vi "App_Main 2.vi"() -> ()   [LabVIEW 2015, in "Application 2.lvlib"]
uses:
  Application 2.lvlib
  Cloud Server/Data Def/Server_Error Handle Method.ctl
  Data Def/App_Subpanel Name.ctl
  Data Def/App_User Event Data.ctl
  Data Def/App_Main Loop Queue Data.ctl
  Data Def/App_Tips Data.ctl
  Cloud Server/Cloud Server.lvlib
panel:
  out "Time":timestamp format="%<%H:%M:%S>T"
  out "Connection?":bool
  out "User Name":string
  out "Login?":bool
  out "Tips":string
  in  "Stop":bool caption="Power"
  in  "Home":bool caption="Menu"
  # "Smart ECG Client"
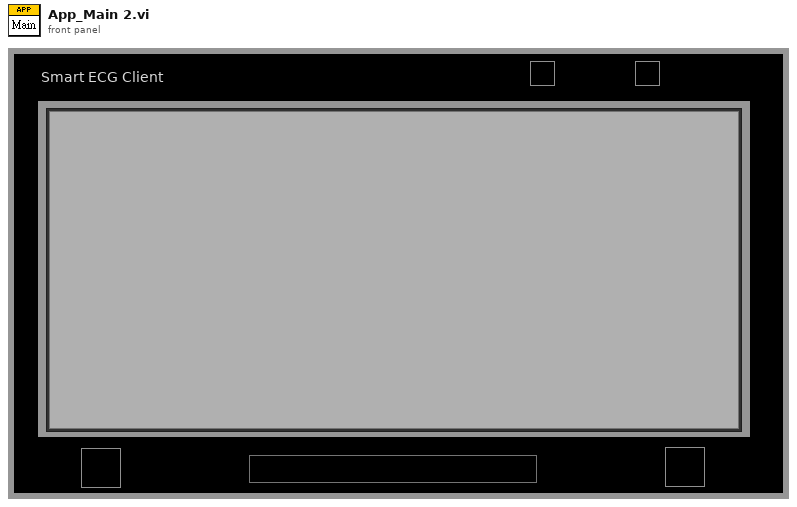
[diagram p1: front panel]
types:
  T1 = typedef "Cloud Server.lvlib/Server_Error Handle Method.ctl" = enum16{"Initialize", "Get Queue Ref.", "Enqueue", "Insert", "Flush", "Release"}
  T2 = typedef "Application 2.lvlib/App_User Event Data.ctl" = cluster{"Command":string, "Data":variant}
  T3 = typedef "Application 2.lvlib/App_Subpanel Name.ctl" = enum16{"Main", "Menu", "User Registering", "User Setting", "Monitor", "Traning Mode", "Query Data", "Connect Setting"}
  T4 = typedef "Application 2.lvlib/App_Main Loop Queue Data.ctl" = cluster{"Command":string, "Data":variant}
  T5 = typedef "Application 2.lvlib/App_Main Data.ctl" = cluster{"VI Refnum":refnum<vi>, "Subpanel":refnum<vi>, "Connection ID":refnum<k5>, "Meta data":T6[], "Main Queue":T8, "User Data":T9}
  T6 = typedef "stm_MetaElement.ctl" = cluster{"Name":T7}
  T7 = typedef "stm_MetaDataElement.ctl" = string
  T8 = typedef "Application 2.lvlib/App_Main Queue.ctl" = cluster{"Main Loop Queue":refnum<queue>}
  T9 = typedef "User Data.ctl" = cluster{"Name":string, "Email":string, "Phone Number":string, "User Picture":u32[][], "Last Login Time":timestamp}
  T10 = typedef "Application 2.lvlib/App_Tips Data.ctl" = cluster{"Tips":string, "BG Color":u32}
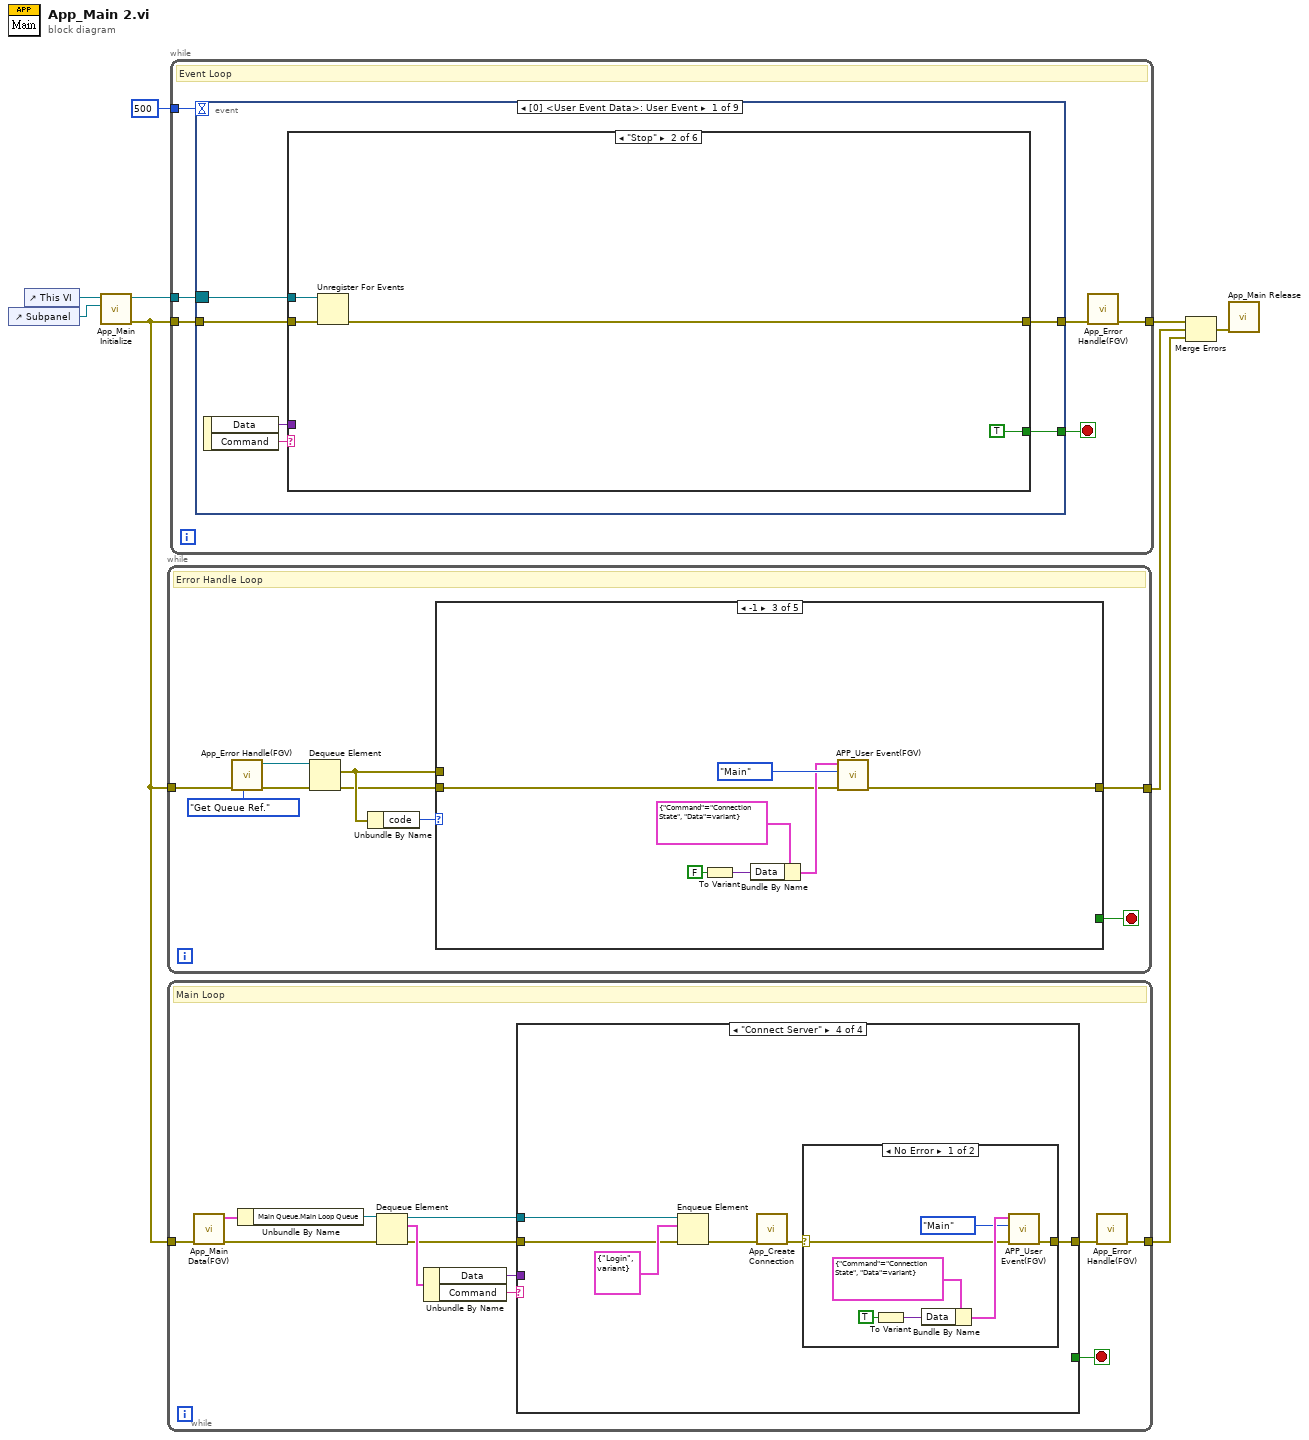
[diagram p0: block diagram]
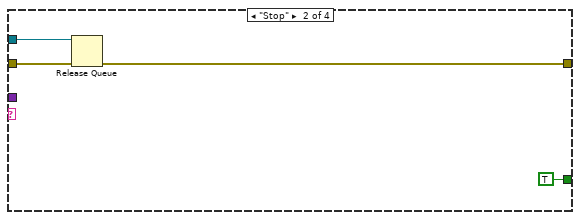
[diagram p3: hidden frame]
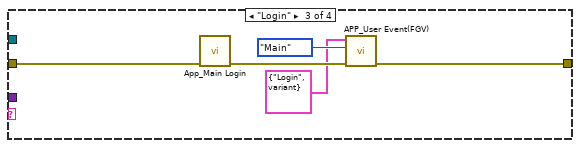
[diagram p4: hidden frame]
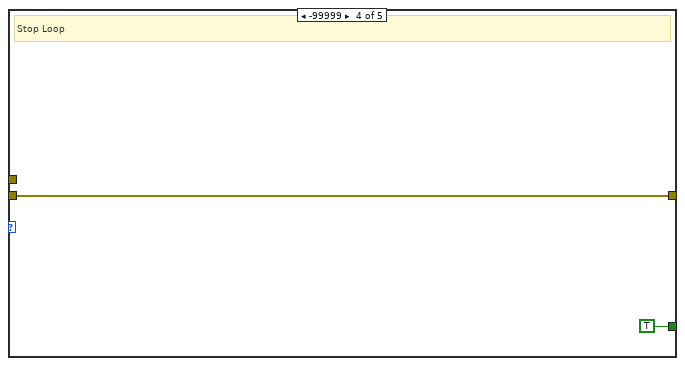
[diagram p8: hidden frame]
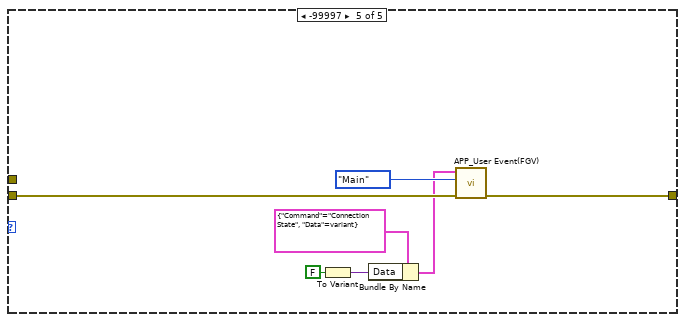
[diagram p9: hidden frame]
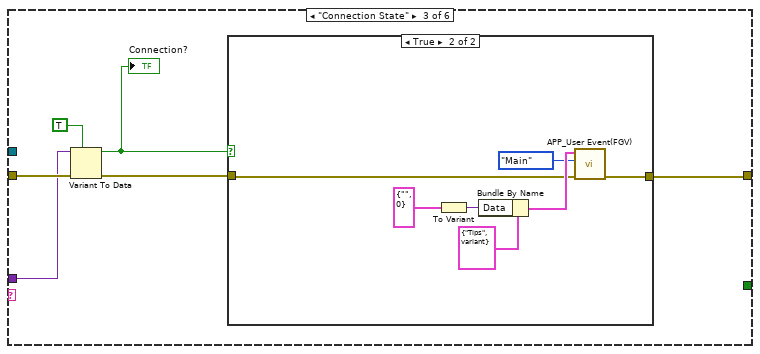
[diagram p11: hidden frame]
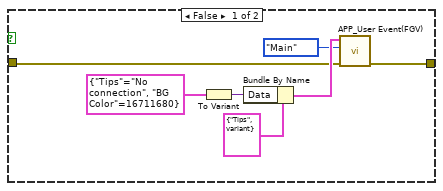
[diagram p12: hidden frame]
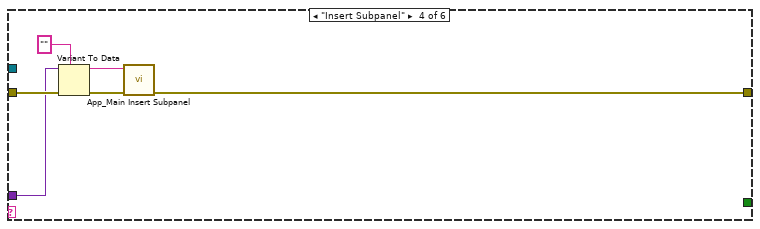
[diagram p13: hidden frame]
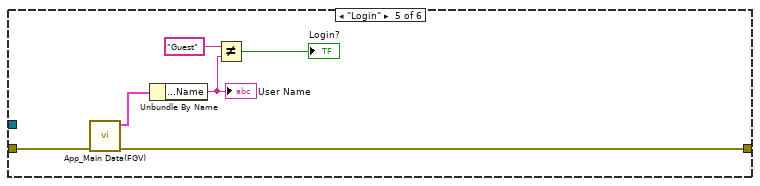
[diagram p14: hidden frame]
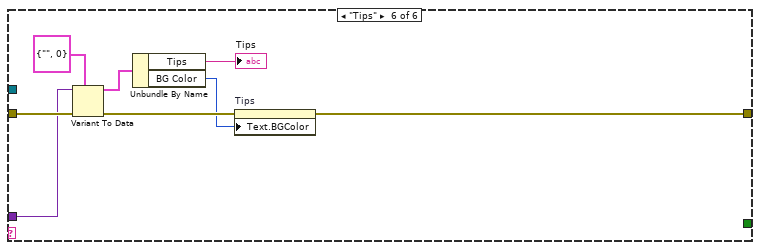
[diagram p15: hidden frame]
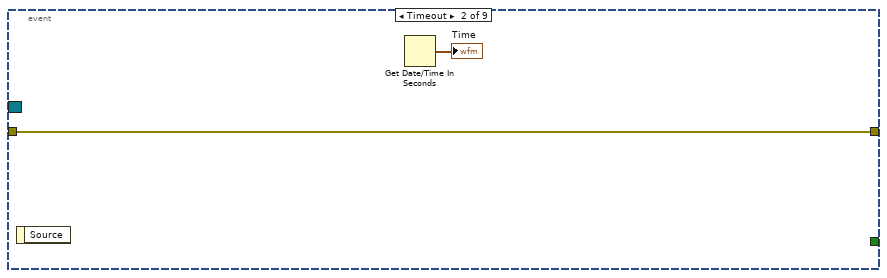
[diagram p16: hidden frame]
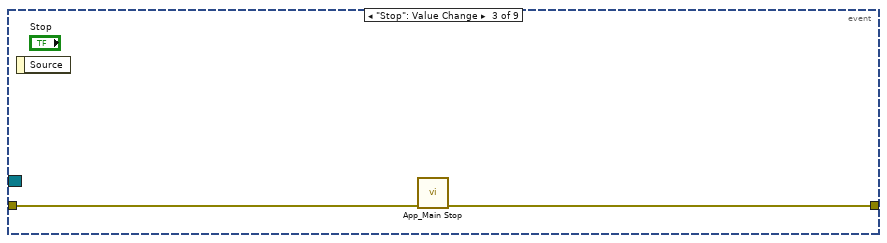
[diagram p17: hidden frame]
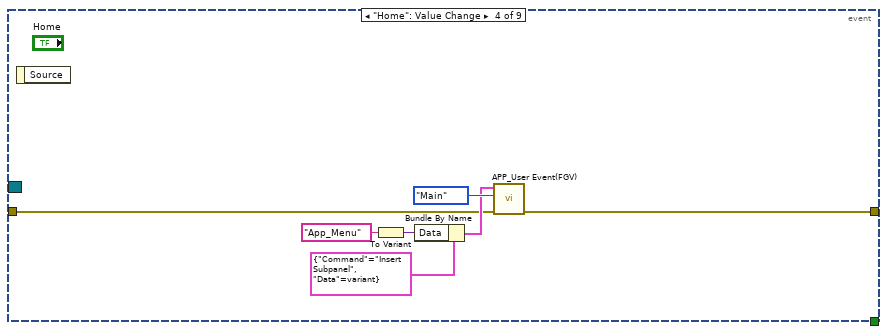
[diagram p18: hidden frame]
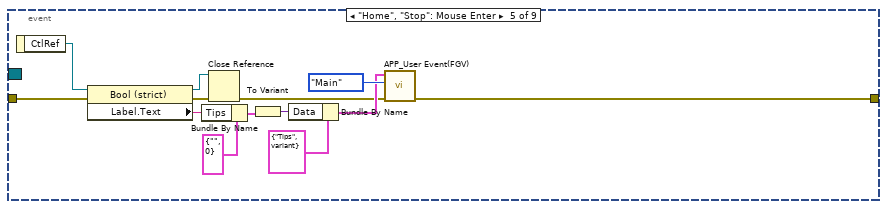
[diagram p19: hidden frame]
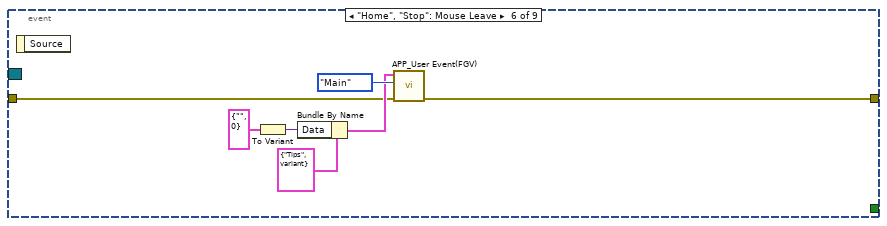
[diagram p20: hidden frame]
diagram:
  n1 = control-ref of="Subpanel"() -> (w7:refnum<vi>)
  n2 = control-ref of="This VI"() -> (w9:refnum<vi>)
  n3 = call "App_Main Initialize.vi"("Subpanel"=w7, "VI Reference"=w9) -> ("error out"=w2:errorcluster, "Event Registration Refnum"=w8:refnum<event-registration>)  [unwired: 8 in]
  n4 = while {
    tunnel: w2 -> [w18]
    tunnel: [w10] -> w4
    stop <- w11 stop-if-true
    # "Error Handle Loop"
    n5 = call "App_Error Handle(FGV).vi"("Error Handle Method(Enqueue)"=Server_Error_Handle_Method."Get Queue Ref.", "error in"=w18) -> ("error out"=w16:errorcluster, "Queue Ref."=w15:refnum<queue>)  [unwired: 8 in]
    n6 = Dequeue Element(queue=w15, error in (no error)=w16) -> (element=w13:errorcluster, error out=w12:errorcluster)  [unwired: 1 in, 2 out]
    n7 = Unbundle By Name(w13) -> ("code"=w14:i32)
    n8 = case shown="-1" w14 {
      tunnel: w13 -> [_ _ _ _ _]
      tunnel: w12 -> [w19 w20 w22 w28 w35]
      tunnel: [_ _ _ TRUE _] -> w11
      tunnel: [w19 w20 w21 w28 w30] -> w10
      frame Default {
        # "Undefine error"
      }
      frame 0 {
        # "No error"
      }
      frame -1 {
        n9 = To Variant(anything=FALSE) -> (Variant=w25:variant)
        n10 = Bundle By Name(cluster=T2 {"Command"="Connection State", "Data"=variant} ("User Event Data"), "Data"=w25) -> (w23:T2)
        n11 = call "APP_User Event(FGV).vi"("error in"=w22, "Subpanel Name"=App_Subpanel_Name."Main", "User Event Data"=w23) -> ("error out"=w21:errorcluster)  [unwired: 7 in, 1 out]
      }
      frame -99999 {
        # "Stop Loop"
      }
      frame -99997 {
        n12 = To Variant(anything=FALSE) -> (Variant=w33:variant)
        n13 = Bundle By Name(cluster=T2 {"Command"="Connection State", "Data"=variant} ("User Event Data"), "Data"=w33) -> (w31:T2)
        n14 = call "APP_User Event(FGV).vi"("error in"=w35, "Subpanel Name"=App_Subpanel_Name."Main", "User Event Data"=w31) -> ("error out"=w30:errorcluster)  [unwired: 7 in, 1 out]
      }
    }
  }
  n15 = while {
    tunnel: w2 -> [w48]
    tunnel: [w39] -> w1
    stop <- w37 stop-if-true
    # "Main Loop"
    n16 = call "App_Main Data(FGV).vi"("error in"=w48) -> ("error out"=w46:errorcluster, "Main Data Out"=w47:T5)  [unwired: 9 in]
    n17 = Unbundle By Name(w47) -> ("Main Queue.Main Loop Queue"=w45:refnum<queue>)
    n18 = Dequeue Element(queue=w45, error in (no error)=w46) -> (queue out=w38:refnum<queue>, element=w44:T4, error out=w41:errorcluster)  [unwired: 1 in, 1 out]
    n19 = Unbundle By Name(w44) -> ("Data"=w42:variant, "Command"=w43:string)
    n20 = case shown="\"Connect Server\"" w43 {
      tunnel: w42 -> [_ _ _ _]
      tunnel: w41 -> [w49 w53 w58 w61]
      tunnel: [w49 w51 w54 w63] -> w40
      tunnel: w38 -> [_ w52 _ w59]
      tunnel: [_ TRUE _ _] -> w37
      frame Default {
      }
      frame "Stop" {
        n21 = Release Queue(queue=w52, error in (no error)=w53) -> (error out=w51:errorcluster)  [unwired: 1 in, 2 out]
      }
      frame "Login" {
        n22 = call "App_Main Login.vi"("error in"=w58) -> ("error out"=w56:errorcluster)  [unwired: 10 in]
        n23 = call "APP_User Event(FGV).vi"("error in"=w56, "Subpanel Name"=App_Subpanel_Name."Main", "User Event Data"=T2 {"Command"="Login", "Data"=variant}) -> ("error out"=w54:errorcluster)  [unwired: 7 in, 1 out]
      }
      frame "Connect Server" {
        n24 = Enqueue Element(queue=w59, element=T4 {"Command"="Login", "Data"=variant}, error in (no error)=w61) -> (error out=w60:errorcluster)  [unwired: 1 in, 2 out]
        n25 = call "App_Create Connection.vi"("error in"=w60) -> ("error out"=w64:errorcluster)  [unwired: 10 in]
        n26 = case shown="No Error" w64 {
          selector: w64 -> [w66 w72]
          tunnel: [w65 w72] -> w63
          frame No Error {
            n27 = To Variant(anything=TRUE) -> (Variant=w69:variant)
            n28 = Bundle By Name(cluster=T2 {"Command"="Connection State", "Data"=variant} ("User Event Data"), "Data"=w69) -> (w71:T2)
            n29 = call "APP_User Event(FGV).vi"("error in"=w66, "Subpanel Name"=App_Subpanel_Name."Main", "User Event Data"=w71) -> ("error out"=w65:errorcluster)  [unwired: 7 in, 1 out]
          }
          frame Error {
          }
        }
      }
    }
    n30 = call "App_Error Handle(FGV).vi"("error in"=w40) -> ("error out"=w39:errorcluster)  [unwired: 9 in, 1 out]
  }
  n31 = while {
    tunnel: w2 -> [w77]
    tunnel: w8 -> [w78]
    tunnel: [w74] -> w5
    tunnel: 500 -> [w73]
    stop <- w76 stop-if-true
    # "Event Loop"
    n32 = event shown="[0] <User Event Data>: User Event" {
      selector: w78 -> [w81 _ _ _ _ _ _ _ _]
      dyn-events: _ -> [_ _ _ _ _ _ _ _ _]
      timeout: w73 -> [_ _ _ _ _ _ _ _ _]
      tunnel: w77 -> [w82 w130 w133 w135 w153 w156 w164 w169 w183]
      tunnel: [w80 w130 w132 w134 w144 w155 w163 w168 w182] -> w75
      tunnel: [w79 _ _ _ _ _ _ _ _] -> w76
      event User Event {
        n33 = event-data() -> ("Data"=w83:variant, "Command"=w84:string)  [unwired: 1 in]
        n34 = case shown="\"Stop\"" w84 {
          tunnel: w83 -> [_ _ w94 w114 _ w128]
          tunnel: w82 -> [w85 w89 w95 w115 w121 w129]
          tunnel: w81 -> [_ w88 _ _ _ _]
          tunnel: [w85 w87 w90 w110 w119 w126] -> w80
          tunnel: [_ TRUE _ _ _ _] -> w79
          frame Default {
          }
          frame "Stop" {
            n35 = Unregister For Events(event registration refnum=w88, error in=w89) -> (error out=w87:errorcluster)
          }
          frame "Connection State" {
            n36 = Variant To Data(error in=w95, type=TRUE, Variant=w94) -> (data=w91:bool, error out=w92:errorcluster)
            "Connection?" <- w91
            n37 = case shown="True" w91 {
              tunnel: w92 -> [w97 w104]
              tunnel: [w96 w103] -> w90
              frame False {
                n38 = To Variant(anything=T10 {"Tips"="No connection", "BG Color"=16711680} ("Tips Data")) -> (Variant=w100:variant)
                n39 = Bundle By Name(cluster=T2 {"Command"="Tips", "Data"=variant} ("User Event Data"), "Data"=w100) -> (w101:T2)
                n40 = call "APP_User Event(FGV).vi"("error in"=w97, "Subpanel Name"=App_Subpanel_Name."Main", "User Event Data"=w101) -> ("error out"=w96:errorcluster)  [unwired: 7 in, 1 out]
              }
              frame True {
                n41 = To Variant(anything=T10 {"Tips"="", "BG Color"=0} ("Tips Data")) -> (Variant=w107:variant)
                n42 = Bundle By Name(cluster=T2 {"Command"="Tips", "Data"=variant} ("User Event Data"), "Data"=w107) -> (w108:T2)
                n43 = call "APP_User Event(FGV).vi"("error in"=w104, "Subpanel Name"=App_Subpanel_Name."Main", "User Event Data"=w108) -> ("error out"=w103:errorcluster)  [unwired: 7 in, 1 out]
              }
            }
          }
          frame "Insert Subpanel" {
            n44 = Variant To Data(error in=w115, type="", Variant=w114) -> (data=w111:string, error out=w112:errorcluster)
            n45 = call "App_Main Insert Subpanel.vi"("error in"=w112, "VI Name"=w111) -> ("error out"=w110:errorcluster)  [unwired: 9 in]
          }
          frame "Login" {
            n46 = call "App_Main Data(FGV).vi"("error in"=w121) -> ("error out"=w119:errorcluster, "Main Data Out"=w120:T5)  [unwired: 9 in]
            n47 = Unbundle By Name(w120) -> ("User Data.Name"=w118:string)
            "User Name" <- w118
            n48 = Not Equal?(x="Guest", y=w118) -> (x != y?=→"Login?":bool)
          }
          frame "Tips" {
            n49 = Variant To Data(error in=w129, type=T10 {"Tips"="", "BG Color"=0} ("Tips Data"), Variant=w128) -> (data=w124:T10, error out=w127:errorcluster)
            n50 = Unbundle By Name(w124) -> ("Tips"=→"Tips":string, "BG Color"=w122:u32)
            n51 = property on="Tips" class="Str"(error in=w127, "Text.BGColor"=w122) -> (error out=w126:errorcluster)  [unwired: 1 in, 1 out]
          }
        }
      }
      event Timeout {
        n52 = event-data() -> ()  [unwired: 1 in, 1 out]
        n53 = Get Date/Time In Seconds() -> (seconds since 1Jan1904=→"Time":timestamp)
      }
      event "Stop": Value Change {
        n54 = event-data() -> ()  [unwired: 1 in, 1 out]
        n55 = call "App_Main Stop.vi"("error in"=w133) -> ("error out"=w132:errorcluster)  [unwired: 10 in]
      }
      event "Home": Value Change {
        n56 = event-data() -> ()  [unwired: 1 in, 1 out]
        n57 = To Variant(anything="App_Menu") -> (Variant=w138:variant)
        n58 = Bundle By Name(cluster=T2 {"Command"="Insert Subpanel", "Data"=variant} ("User Event Data"), "Data"=w138) -> (w136:T2)
        n59 = call "APP_User Event(FGV).vi"("error in"=w135, "Subpanel Name"=App_Subpanel_Name."Main", "User Event Data"=w136) -> ("error out"=w134:errorcluster)  [unwired: 7 in, 1 out]
      }
      event "Home", "Stop": Mouse Enter {
        n60 = event-data() -> ("CtlRef"=w152:refnum<vi>)  [unwired: 1 in]
        n61 = property class="Bool (strict)"(reference=w152, error in=w153) -> (reference out=w146:refnum<vi>, error out=w147:errorcluster, "Label.Text"=w142:string)
        n62 = Bundle By Name(cluster=T10 {"Tips"="", "BG Color"=0} ("Tips Data"), "Tips"=w142) -> (w143:T10)
        n63 = Close Reference(reference=w146, error in (no error)=w147) -> (error out=w145:errorcluster)
        n64 = To Variant(anything=w143) -> (Variant=w149:variant)
        n65 = Bundle By Name(cluster=T2 {"Command"="Tips", "Data"=variant} ("User Event Data"), "Data"=w149) -> (w148:T2)
        n66 = call "APP_User Event(FGV).vi"("error in"=w145, "Subpanel Name"=App_Subpanel_Name."Main", "User Event Data"=w148) -> ("error out"=w144:errorcluster)  [unwired: 7 in, 1 out]
      }
      event "Home", "Stop": Mouse Leave {
        n67 = event-data() -> ()  [unwired: 1 in, 1 out]
        n68 = To Variant(anything=T10 {"Tips"="", "BG Color"=0} ("Tips Data")) -> (Variant=w158:variant)
        n69 = Bundle By Name(cluster=T2 {"Command"="Tips", "Data"=variant} ("User Event Data"), "Data"=w158) -> (w157:T2)
        n70 = call "APP_User Event(FGV).vi"("error in"=w156, "Subpanel Name"=App_Subpanel_Name."Main", "User Event Data"=w157) -> ("error out"=w155:errorcluster)  [unwired: 7 in, 1 out]
      }
      event "Connection?": Mouse Up {
        n71 = event-data() -> ()  [unwired: 1 in, 1 out]
        n72 = To Variant(anything="App_Connect Setting") -> (Variant=w162:variant)
        n73 = Bundle By Name(cluster=T2 {"Command"="Insert Subpanel", "Data"=variant} ("User Event Data"), "Data"=w162) -> (w165:T2)
        n74 = call "APP_User Event(FGV).vi"("error in"=w164, "Subpanel Name"=App_Subpanel_Name."Main", "User Event Data"=w165) -> ("error out"=w163:errorcluster)  [unwired: 7 in, 1 out]
      }
      event "Login?": Mouse Up {
        n75 = event-data() -> ()  [unwired: 1 in, 1 out]
        n76 = call "App_Main Data(FGV).vi"("error in"=w169) -> ("error out"=w176:errorcluster, "Main Data Out"=w175:T5)  [unwired: 9 in]
        n77 = Unbundle By Name(w175) -> ("User Data.Name"=w173:string)
        n78 = Not Equal?(x="Guest", y=w173) -> (x != y?=w172:bool)
        n79 = Select(t="App_User Setting", s=w172, f="App_User Registering") -> (s? t:f=w177:string)
        n80 = To Variant(anything=w177) -> (Variant=w180:variant)
        n81 = Bundle By Name(cluster=T2 {"Command"="Insert Subpanel", "Data"=variant} ("User Event Data"), "Data"=w180) -> (w178:T2)
        n82 = call "APP_User Event(FGV).vi"("error in"=w176, "Subpanel Name"=App_Subpanel_Name."Main", "User Event Data"=w178) -> ("error out"=w168:errorcluster)  [unwired: 7 in, 1 out]
      }
      event Panel Close? {
        n83 = event-data() -> ()  [unwired: 1 in, 1 out]
        n84 = call "App_Main Stop.vi"("error in"=w183) -> ("error out"=w182:errorcluster)  [unwired: 10 in]
        n85 = event-data("Discard?"=TRUE) -> ()  [unwired: 1 in, 1 out]
      }
    }
    n86 = call "App_Error Handle(FGV).vi"("error in"=w75) -> ("error out"=w74:errorcluster)  [unwired: 9 in, 1 out]
  }
  n87 = Merge Errors(w5, w4, w1) -> (w3:errorcluster)
  n88 = call "App_Main Release.vi"("error in"=w3) -> ()  [unwired: 10 in, 1 out]
